vi "Configurations.vi"(8 "Mode":T4) -> (0 "Configuration":T1={"Mode"="", "InstrumentMode"={"MainDAQ_Selector"=enum."None", "LaserCtrlMethod"=enum."SRS_DG535", "InstruMode"=enum."fsLDPI"}, "CommuniationSettings"={"SDG_II"="", "DG535"="", "BNC565"="", "EPM2000"="", "NI-DAQmx"="", "Micos"={"Simulation"=FALSE, "ComPort"="", "Serial Config"={"Baud Rate"=0, "Parity"=0, "Data Bits"=0, "Stop Bits"=0, "Flow Control"=0}, "#Axis"=0}, "ESP300"={"Simulation"=FALSE, "ComPort"="", "Serial Config"={"Baud Rate"=0, "Parity"=0, "Data Bits"=0, "Stop Bits"=0, "Flow Control"=0}, "#Axis"=0}}, "DG535"={"Trigger"={"Trigger Mode"=enum."Internal", "Internal/Burst Rate"=0.0, "External  Level"=0.0, "Impedance"=FALSE, "Slope"=FALSE}, "Delays"=[], "Output"=[]}, "Gage_Config"={"Acquisition"={"Sample Rate"=0.0, "Mode"=0, "Start (0)"=0.0, "Depth"=0.0, "Segment Size"=0.0, "Trigger Delay"=0.0, "Trigger Timeout"=0.0, "Trigger Holdoff"=0.0, "Clock mode"=enum."Internal"}, "Channels"=[], "Trigger"={"Slope"=0, "Level"=0, "Source"=0, "External Range"=0, "External Coupling"=0, "External"=FALSE, "Disable"=FALSE, "External Impedance"=0}, "Mode(Gage)"=enum."Normal"}, "AnalogDisc_Config"={"Acqusition"={"Freq(Hz,SampleRate)"=0.0, "BufferSize"=0, "Mode"=enum."Single", "RecordLength(s)"=0.0}, "Channels"=[], "Trigger"={"TriggerSource"=enum."None", "Timeout(s)"=0.0, "Holdoff(s)"=0.0, "Position/Delay(s)"=0.0}, "AnalogTrigger"={"Channel"=0, "Polarity"=enum."Rising", "Type"=enum."Edge", "Level(V)"=0.0, "Filter"=enum."Decimate", "Hysterisis(V)"=0.0}}, "Micos"={"Velocity"=0.0, "Acceleration"=0.0}, "ESP300"={"Velocity"=[], "Acceleration"=[]}, "EPM2000"={"Factor(A)"=0.0, "Factor(B)"=0.0}, "ProcessMethod"={"TopLine"=0.0, "Threshold"=0.0, "Baseline"=0.0, "ZeroOffset"=0.0, "Processing Mode"=enum."None"}, "Timing(LDPI)"={"Delay(PI)"=0.0, "Delay(Rejection)"=0.0, "NoDelayOffset"=0.0, "RepRate(Hz)"=0.0}, "Cali."=[0.0707, 0.16163, 0.02539], "BNC_Config"={"System"={"Rep.Rate"=1000.0, "Sys Ext Mode"=enum."Triggered", "Mode"=enum."Single Shot"}, "Channels"=[]}} {"Cali." format="%#.6f"; "Timing(LDPI)"."Delay(PI)" format="%#_6p"; "Timing(LDPI)"."Delay(Rejection)" format="%#_6p"; "Timing(LDPI)"."NoDelayOffset" format="%#_6p"; "DG535"."Trigger"."External  Level" min=-2.56 max=2.56 format="%.2f"; "DG535"."Trigger"."Internal/Burst Rate" min=0.001 max=1000000.0 format="%.3f"; "DG535"."Delays"."Delay" format="%#_6p"; "DG535"."Output"."Offset" min=-3.0 max=4.0 format="%.2f"; "DG535"."Output"."Amplitude" min=-3.0 max=4.0 format="%.2f"; "ProcessMethod"."Threshold" format="%#_6p"; "Gage_Config"."Trigger"."External Impedance" items=["50 Ohm", "HiZ"]; "Gage_Config"."Trigger"."External Coupling" items=["DC", "AC"]; "Gage_Config"."Trigger"."External Range" min=2000 max=10000 step=8000; "Gage_Config"."Trigger"."Slope" items=["Rising", "Falling"]; "Gage_Config"."Trigger"."Level" min=-100 max=100; "Gage_Config"."Trigger"."Source" min=0 max=64 step=1; "Gage_Config"."Channels"."Impedance" min=50 max=1000000 step=999950; "Gage_Config"."Channels"."Coupling" items=["DC", "AC"]; "Gage_Config"."Acquisition"."Segment Size" min=256.0 step=128.0; "Gage_Config"."Acquisition"."Trigger Delay" min=0.0 step=128.0; "Gage_Config"."Acquisition"."Trigger Timeout" format="%.0p"; "Gage_Config"."Acquisition"."Trigger Holdoff" min=0.0 step=128.0; "Gage_Config"."Acquisition"."Depth" min=256.0 step=128.0; "Gage_Config"."Acquisition"."Mode" items=["Single", "Dual", "Quad", "Octal"]; "Gage_Config"."Acquisition"."Sample Rate" format="%.0p"; "AnalogDisc_Config"."AnalogTrigger"."Level(V)" format="%#_6p"; "AnalogDisc_Config"."AnalogTrigger"."Hysterisis(V)" format="%#_6p"; "AnalogDisc_Config"."Acqusition"."RecordLength(s)" format="%#_6p"; "AnalogDisc_Config"."Acqusition"."Freq(Hz,SampleRate)" format="%#_6p"; "AnalogDisc_Config"."Trigger"."Position/Delay(s)" format="%#_6p"; "AnalogDisc_Config"."Trigger"."Holdoff(s)" format="%#_6p"; "AnalogDisc_Config"."Trigger"."Timeout(s)" format="%#_6p"})   [LabVIEW 2013]
uses:
  ControlDef/InstrumentConfiguration.ctl
  ControlDef/MainDAQ_Selector.ctl
  ControlDef/LaserCtrl_Method.ctl
  ControlDef/InstruMode_Typedef.ctl
  <instrlib>/DG535/Command/Set Trigger.ctl
  <instrlib>/DG535/Command/DG535_TriggerMode.ctl
  <instrlib>/DG535/Command/Set Delay.ctl
  <instrlib>/DG535/Command/DG535_Channel.ctl
  <instrlib>/DG535/Command/Set Output.ctl
  <instrlib>/DG535/Command/DG535_Output.ctl
  <instrlib>/GageLv_uic/VI/Gage_Configs.ctl
  <instrlib>/AnalogDiscSDKLv/VIs/DWF_AnalogIn_Configurations.ctl
  <instrlib>/AnalogDiscSDKLv/VIs/DWF_AcqMode.ctl
  <instrlib>/AnalogDiscSDKLv/VIs/DWF_Filter.ctl
  <instrlib>/AnalogDiscSDKLv/VIs/DWF_TrigSrc.ctl
  <instrlib>/AnalogDiscSDKLv/VIs/DWF_TrigCond.ctl
  <instrlib>/AnalogDiscSDKLv/VIs/DWF_TrigType.ctl
  ControlDef/ProcessingMode.ctl
  <instrlib>/BNC/Public/BNC_Configs.ctl
  ControlDef/InstrumentSpecificControls/UIC-AToF/InitializationParams_BNC565_2Ch_AToF.ctl
  Hardware/BNC(QuantumComposers)/Command/Set C-Input.ctl
  Hardware/BNC(QuantumComposers)/Command/Set C-Mode.ctl
  Hardware/BNC(QuantumComposers)/Command/Set C-Output.ctl
  Hardware/BNC(QuantumComposers)/Command/Set C-Enable.ctl
  <instrlib>/DG535/SRS_DG535_Lib.lvlib
  <instrlib>/GageLv_uic/Gage.lvlib
  <instrlib>/AnalogDiscSDKLv/AnalogDiscSDKLv.lvlib
panel:
  in  "GetConfigurations":T1[](array[typedef])=[{"Mode"="fsLDPI", "InstrumentMode"={"MainDAQ_Selector"=enum."Gage", "LaserCtrlMethod"=enum."SDG_II", "InstruMode"=enum."fsLDPI"}, "CommuniationSettings"={"SDG_II"="COM6", "DG535"="GPIB0::5::INSTR", "BNC565"="", "EPM2000"="COM5", "NI-DAQmx"="", "Micos"={"Simulation"=FALSE, "ComPort"="COM3", "Serial Config"={"Baud Rate"=115200, "Parity"=0, "Data Bits"=8, "Stop Bits"=10, "Flow Control"=0}, "#Axis"=3}, "ESP300"={"Simulation"=FALSE, "ComPort"="COM7", "Serial Config"={"Baud Rate"=19200, "Parity"=0, "Data Bits"=8, "Stop Bits"=10, "Flow Control"=0}, "#Axis"=3}}, "DG535"={"Trigger"={"Trigger Mode"=enum."External", "Internal/Burst Rate"=10.0, "External  Level"=1.5, "Impedance"=TRUE, "Slope"=FALSE}, "Delays"=[{"Channel"=enum."A Output", "Sync To"=enum."T0 Output", "Delay"=0.0998095}, {"Channel"=enum."B Output", "Sync To"=enum."A Output", "Delay"=2.5e-05}, {"Channel"=enum."C Output", "Sync To"=enum."T0 Output", "Delay"=0.0}, {"Channel"=enum."D Output", "Sync To"=enum."T0 Output", "Delay"=2.3e-05}, {"Channel"=enum."Trigger Input", "Sync To"=enum."T0 Output", "Delay"=0.0}], "Output"=[{"Channel"=enum."A Output", "Level"=enum."TTL", "Load"=TRUE, "Polarity"=TRUE, "Amplitude"=1.0, "Offset"=0.0}, {"Channel"=enum."B Output", "Level"=enum."TTL", "Load"=FALSE, "Polarity"=TRUE, "Amplitude"=1.0, "Offset"=0.0}, {"Channel"=enum."C Output", "Level"=enum."TTL", "Load"=TRUE, "Polarity"=FALSE, "Amplitude"=1.0, "Offset"=0.0}, {"Channel"=enum."D Output", "Level"=enum."TTL", "Load"=TRUE, "Polarity"=FALSE, "Amplitude"=1.0, "Offset"=0.0}, {"Channel"=enum."T0 Output", "Level"=enum."TTL", "Load"=FALSE, "Polarity"=TRUE, "Amplitude"=1.0, "Offset"=0.0}, {"Channel"=enum."AB Output", "Level"=enum."TTL", "Load"=TRUE, "Polarity"=FALSE, "Amplitude"=1.0, "Offset"=0.0}, {"Channel"=enum."CD Output", "Level"=enum."TTL", "Load"=FALSE, "Polarity"=FALSE, "Amplitude"=1.0, "Offset"=0.0}]}, "Gage_Config"={"Acquisition"={"Sample Rate"=500000000.0, "Mode"=0, "Start (0)"=0.0, "Depth"=32768.0, "Segment Size"=32768.0, "Trigger Delay"=0.0, "Trigger Timeout"=-1.0, "Trigger Holdoff"=0.0, "Clock mode"=enum."Internal"}, "Channels"=[{"Coupling"=1, "Differential Input"=FALSE, "Direct-to-ADC"=FALSE, "Range"=2000, "Impedance"=50, "DC Offset"=0, "Filter"=0}], "Trigger"={"Slope"=1, "Level"=25, "Source"=0, "External Range"=10000, "External Coupling"=0, "External"=TRUE, "Disable"=FALSE, "External Impedance"=0}, "Mode(Gage)"=enum."Continuous"}, "AnalogDisc_Config"={"Acqusition"={"Freq(Hz,SampleRate)"=10000000.0, "BufferSize"=8192, "Mode"=enum."Single", "RecordLength(s)"=8192.0}, "Channels"=[], "Trigger"={"TriggerSource"=enum."None", "Timeout(s)"=0.0, "Holdoff(s)"=1e-06, "Position/Delay(s)"=0.0}, "AnalogTrigger"={"Channel"=0, "Polarity"=enum."Rising", "Type"=enum."Pulse", "Level(V)"=0.0, "Filter"=enum."Decimate", "Hysterisis(V)"=0.0}}, "Micos"={"Velocity"=10.0, "Acceleration"=20.0}, "ESP300"={"Velocity"=[0.2, 0.2, 2.0], "Acceleration"=[0.8, 0.8, 0.8]}, "EPM2000"={"Factor(A)"=1.0, "Factor(B)"=1.0}, "ProcessMethod"={"TopLine"=1.0, "Threshold"=0.01, "Baseline"=0.0, "ZeroOffset"=0.0, "Processing Mode"=enum."Drop by Threshold"}, "Timing(LDPI)"={"Delay(PI)"=2.5e-05, "Delay(Rejection)"=-2e-06, "NoDelayOffset"=0.0998095, "RepRate(Hz)"=10.0}, "Cali."=[0.0707, 0.16163, 0.02539], "BNC_Config"={"System"={"Rep.Rate"=1000.0, "Sys Ext Mode"=enum."Triggered", "Mode"=enum."Single Shot"}, "Channels"=[]}}, {"Mode"="nsLDPI", "InstrumentMode"={"MainDAQ_Selector"=enum."Gage", "LaserCtrlMethod"=enum."SDG_II", "InstruMode"=enum."nsLDPI"}, "CommuniationSettings"={"SDG_II"="", "DG535"="GPIB0::5::INSTR", "BNC565"="", "EPM2000"="COM5", "NI-DAQmx"="", "Micos"={"Simulation"=FALSE, "ComPort"="COM3", "Serial Config"={"Baud Rate"=115200, "Parity"=0, "Data Bits"=8, "Stop Bits"=10, "Flow Control"=0}, "#Axis"=3}, "ESP300"={"Simulation"=FALSE, "ComPort"="COM7", "Serial Config"={"Baud Rate"=19200, "Parity"=0, "Data Bits"=8, "Stop Bits"=10, "Flow Control"=0}, "#Axis"=3}}, "DG535"={"Trigger"={"Trigger Mode"=enum."External", "Internal/Burst Rate"=10.0, "External  Level"=1.5, "Impedance"=TRUE, "Slope"=FALSE}, "Delays"=[{"Channel"=enum."A Output", "Sync To"=enum."T0 Output", "Delay"=0.0998095}, {"Channel"=enum."B Output", "Sync To"=enum."A Output", "Delay"=2.5e-05}, {"Channel"=enum."C Output", "Sync To"=enum."T0 Output", "Delay"=0.0}, {"Channel"=enum."D Output", "Sync To"=enum."T0 Output", "Delay"=2.3e-05}, {"Channel"=enum."Trigger Input", "Sync To"=enum."T0 Output", "Delay"=0.0}], "Output"=[{"Channel"=enum."A Output", "Level"=enum."TTL", "Load"=TRUE, "Polarity"=TRUE, "Amplitude"=1.0, "Offset"=0.0}, {"Channel"=enum."B Output", "Level"=enum."TTL", "Load"=FALSE, "Polarity"=TRUE, "Amplitude"=1.0, "Offset"=0.0}, {"Channel"=enum."C Output", "Level"=enum."TTL", "Load"=TRUE, "Polarity"=FALSE, "Amplitude"=1.0, "Offset"=0.0}, {"Channel"=enum."D Output", "Level"=enum."TTL", "Load"=TRUE, "Polarity"=FALSE, "Amplitude"=1.0, "Offset"=0.0}, {"Channel"=enum."T0 Output", "Level"=enum."TTL", "Load"=FALSE, "Polarity"=TRUE, "Amplitude"=1.0, "Offset"=0.0}, {"Channel"=enum."AB Output", "Level"=enum."TTL", "Load"=TRUE, "Polarity"=FALSE, "Amplitude"=1.0, "Offset"=0.0}, {"Channel"=enum."CD Output", "Level"=enum."TTL", "Load"=FALSE, "Polarity"=FALSE, "Amplitude"=1.0, "Offset"=0.0}]}, "Gage_Config"={"Acquisition"={"Sample Rate"=500000000.0, "Mode"=0, "Start (0)"=0.0, "Depth"=32768.0, "Segment Size"=32768.0, "Trigger Delay"=0.0, "Trigger Timeout"=-1.0, "Trigger Holdoff"=0.0, "Clock mode"=enum."Internal"}, "Channels"=[{"Coupling"=1, "Differential Input"=FALSE, "Direct-to-ADC"=FALSE, "Range"=2000, "Impedance"=50, "DC Offset"=0, "Filter"=0}], "Trigger"={"Slope"=1, "Level"=25, "Source"=0, "External Range"=10000, "External Coupling"=0, "External"=TRUE, "Disable"=FALSE, "External Impedance"=0}, "Mode(Gage)"=enum."Continuous"}, "AnalogDisc_Config"={"Acqusition"={"Freq(Hz,SampleRate)"=10000000.0, "BufferSize"=8192, "Mode"=enum."Single", "RecordLength(s)"=8192.0}, "Channels"=[], "Trigger"={"TriggerSource"=enum."None", "Timeout(s)"=0.0, "Holdoff(s)"=1e-06, "Position/Delay(s)"=0.0}, "AnalogTrigger"={"Channel"=0, "Polarity"=enum."Rising", "Type"=enum."Pulse", "Level(V)"=0.0, "Filter"=enum."Decimate", "Hysterisis(V)"=0.0}}, "Micos"={"Velocity"=10.0, "Acceleration"=20.0}, "ESP300"={"Velocity"=[0.2, 0.2, 0.2], "Acceleration"=[0.8, 0.8, 0.8]}, "EPM2000"={"Factor(A)"=1.0, "Factor(B)"=1.0}, "ProcessMethod"={"TopLine"=1.0, "Threshold"=0.01, "Baseline"=0.0, "ZeroOffset"=0.0, "Processing Mode"=enum."Drop by Threshold"}, "Timing(LDPI)"={"Delay(PI)"=2.5e-05, "Delay(Rejection)"=-2e-06, "NoDelayOffset"=0.0001766, "RepRate(Hz)"=10.0}, "Cali."=[0.0707, 0.16163, 0.02539], "BNC_Config"={"System"={"Rep.Rate"=1000.0, "Sys Ext Mode"=enum."Triggered", "Mode"=enum."Single Shot"}, "Channels"=[]}}, {"Mode"="nsLD-fsPI", "InstrumentMode"={"MainDAQ_Selector"=enum."Gage", "LaserCtrlMethod"=enum."SDG_II", "InstruMode"=enum."nsLD-fsPI"}, "CommuniationSettings"={"SDG_II"="COM6", "DG535"="GPIB0::5::INSTR", "BNC565"="", "EPM2000"="COM5", "NI-DAQmx"="", "Micos"={"Simulation"=FALSE, "ComPort"="COM3", "Serial Config"={"Baud Rate"=115200, "Parity"=0, "Data Bits"=8, "Stop Bits"=10, "Flow Control"=0}, "#Axis"=3}, "ESP300"={"Simulation"=FALSE, "ComPort"="COM7", "Serial Config"={"Baud Rate"=19200, "Parity"=0, "Data Bits"=8, "Stop Bits"=10, "Flow Control"=0}, "#Axis"=3}}, "DG535"={"Trigger"={"Trigger Mode"=enum."External", "Internal/Burst Rate"=1000.0, "External  Level"=1.5, "Impedance"=TRUE, "Slope"=FALSE}, "Delays"=[{"Channel"=enum."A Output", "Sync To"=enum."T0 Output", "Delay"=0.0009859}, {"Channel"=enum."B Output", "Sync To"=enum."A Output", "Delay"=-2e-05}, {"Channel"=enum."C Output", "Sync To"=enum."T0 Output", "Delay"=5e-05}, {"Channel"=enum."D Output", "Sync To"=enum."T0 Output", "Delay"=0.000998}, {"Channel"=enum."Trigger Input", "Sync To"=enum."T0 Output", "Delay"=0.0}], "Output"=[{"Channel"=enum."A Output", "Level"=enum."TTL", "Load"=TRUE, "Polarity"=TRUE, "Amplitude"=1.0, "Offset"=0.0}, {"Channel"=enum."B Output", "Level"=enum."TTL", "Load"=TRUE, "Polarity"=TRUE, "Amplitude"=1.0, "Offset"=0.0}, {"Channel"=enum."C Output", "Level"=enum."TTL", "Load"=TRUE, "Polarity"=FALSE, "Amplitude"=1.0, "Offset"=0.0}, {"Channel"=enum."D Output", "Level"=enum."TTL", "Load"=TRUE, "Polarity"=FALSE, "Amplitude"=1.0, "Offset"=0.0}, {"Channel"=enum."T0 Output", "Level"=enum."TTL", "Load"=TRUE, "Polarity"=TRUE, "Amplitude"=1.0, "Offset"=0.0}, {"Channel"=enum."AB Output", "Level"=enum."TTL", "Load"=TRUE, "Polarity"=FALSE, "Amplitude"=1.0, "Offset"=0.0}, {"Channel"=enum."CD Output", "Level"=enum."TTL", "Load"=FALSE, "Polarity"=FALSE, "Amplitude"=1.0, "Offset"=0.0}]}, "Gage_Config"={"Acquisition"={"Sample Rate"=500000000.0, "Mode"=0, "Start (0)"=0.0, "Depth"=32768.0, "Segment Size"=32768.0, "Trigger Delay"=0.0, "Trigger Timeout"=-1.0, "Trigger Holdoff"=0.0, "Clock mode"=enum."Internal"}, "Channels"=[{"Coupling"=1, "Differential Input"=FALSE, "Direct-to-ADC"=FALSE, "Range"=2000, "Impedance"=50, "DC Offset"=0, "Filter"=0}], "Trigger"={"Slope"=1, "Level"=25, "Source"=0, "External Range"=10000, "External Coupling"=0, "External"=TRUE, "Disable"=FALSE, "External Impedance"=0}, "Mode(Gage)"=enum."Continuous"}, "AnalogDisc_Config"={"Acqusition"={"Freq(Hz,SampleRate)"=10000000.0, "BufferSize"=8192, "Mode"=enum."Single", "RecordLength(s)"=8192.0}, "Channels"=[], "Trigger"={"TriggerSource"=enum."None", "Timeout(s)"=0.0, "Holdoff(s)"=1e-06, "Position/Delay(s)"=0.0}, "AnalogTrigger"={"Channel"=0, "Polarity"=enum."Rising", "Type"=enum."Edge", "Level(V)"=0.0, "Filter"=enum."Decimate", "Hysterisis(V)"=0.0}}, "Micos"={"Velocity"=10.0, "Acceleration"=20.0}, "ESP300"={"Velocity"=[0.2, 0.2, 2.0], "Acceleration"=[0.8, 0.8, 0.8]}, "EPM2000"={"Factor(A)"=1.0, "Factor(B)"=1.0}, "ProcessMethod"={"TopLine"=1.0, "Threshold"=0.01, "Baseline"=0.0, "ZeroOffset"=0.0, "Processing Mode"=enum."Drop by Threshold"}, "Timing(LDPI)"={"Delay(PI)"=2.5e-05, "Delay(Rejection)"=-2e-06, "NoDelayOffset"=0.0009859, "RepRate(Hz)"=1000.0}, "Cali."=[0.0707, 0.16163, 0.02539], "BNC_Config"={"System"={"Rep.Rate"=1000.0, "Sys Ext Mode"=enum."Triggered", "Mode"=enum."Single Shot"}, "Channels"=[]}}, {"Mode"="GenericTOF", "InstrumentMode"={"MainDAQ_Selector"=enum."Gage", "LaserCtrlMethod"=enum."BNC", "InstruMode"=enum."GenericTOF"}, "CommuniationSettings"={"SDG_II"="", "DG535"="", "BNC565"="COM4", "EPM2000"="", "NI-DAQmx"="", "Micos"={"Simulation"=FALSE, "ComPort"="COM3", "Serial Config"={"Baud Rate"=57600, "Parity"=0, "Data Bits"=8, "Stop Bits"=10, "Flow Control"=0}, "#Axis"=3}, "ESP300"={"Simulation"=TRUE, "ComPort"="", "Serial Config"={"Baud Rate"=19200, "Parity"=0, "Data Bits"=8, "Stop Bits"=10, "Flow Control"=0}, "#Axis"=3}}, "DG535"={"Trigger"={"Trigger Mode"=enum."Internal", "Internal/Burst Rate"=200.0, "External  Level"=1.5, "Impedance"=TRUE, "Slope"=FALSE}, "Delays"=[], "Output"=[]}, "Gage_Config"={"Acquisition"={"Sample Rate"=200000000.0, "Mode"=0, "Start (0)"=0.0, "Depth"=16384.0, "Segment Size"=16384.0, "Trigger Delay"=0.0, "Trigger Timeout"=-1.0, "Trigger Holdoff"=0.0, "Clock mode"=enum."Internal"}, "Channels"=[{"Coupling"=0, "Differential Input"=FALSE, "Direct-to-ADC"=FALSE, "Range"=2000, "Impedance"=50, "DC Offset"=0, "Filter"=0}], "Trigger"={"Slope"=1, "Level"=25, "Source"=0, "External Range"=10000, "External Coupling"=0, "External"=TRUE, "Disable"=FALSE, "External Impedance"=0}, "Mode(Gage)"=enum."Continuous"}, "AnalogDisc_Config"={"Acqusition"={"Freq(Hz,SampleRate)"=10000000.0, "BufferSize"=8192, "Mode"=enum."Single", "RecordLength(s)"=8192.0}, "Channels"=[], "Trigger"={"TriggerSource"=enum."None", "Timeout(s)"=0.0, "Holdoff(s)"=1e-06, "Position/Delay(s)"=0.0}, "AnalogTrigger"={"Channel"=0, "Polarity"=enum."Rising", "Type"=enum."Pulse", "Level(V)"=0.0, "Filter"=enum."Decimate", "Hysterisis(V)"=0.0}}, "Micos"={"Velocity"=10.0, "Acceleration"=20.0}, "ESP300"={"Velocity"=[], "Acceleration"=[]}, "EPM2000"={"Factor(A)"=1.0, "Factor(B)"=1.0}, "ProcessMethod"={"TopLine"=1.0, "Threshold"=0.01, "Baseline"=0.0, "ZeroOffset"=0.0, "Processing Mode"=enum."Drop by Threshold"}, "Timing(LDPI)"={"Delay(PI)"=0.0, "Delay(Rejection)"=0.0, "NoDelayOffset"=0.0, "RepRate(Hz)"=50.0}, "Cali."=[0.0, 1.0, 0.0], "BNC_Config"={"System"={"Rep.Rate"=1000.0, "Sys Ext Mode"=enum."Triggered", "Mode"=enum."Single Shot"}, "Channels"=[]}}, {"Mode"="BeamProfiling", "InstrumentMode"={"MainDAQ_Selector"=enum."AnalogDisc", "LaserCtrlMethod"=enum."SRS_DG535", "InstruMode"=enum."GenericTOF"}, "CommuniationSettings"={"SDG_II"="", "DG535"="GPIB0::5::INSTR", "BNC565"="", "EPM2000"="", "NI-DAQmx"="", "Micos"={"Simulation"=TRUE, "ComPort"="", "Serial Config"={"Baud Rate"=57600, "Parity"=0, "Data Bits"=8, "Stop Bits"=10, "Flow Control"=0}, "#Axis"=3}, "ESP300"={"Simulation"=FALSE, "ComPort"="COM1", "Serial Config"={"Baud Rate"=19200, "Parity"=0, "Data Bits"=8, "Stop Bits"=10, "Flow Control"=0}, "#Axis"=3}}, "DG535"={"Trigger"={"Trigger Mode"=enum."External", "Internal/Burst Rate"=50.0, "External  Level"=1.5, "Impedance"=TRUE, "Slope"=FALSE}, "Delays"=[], "Output"=[]}, "Gage_Config"={"Acquisition"={"Sample Rate"=125000000.0, "Mode"=0, "Start (0)"=0.0, "Depth"=16384.0, "Segment Size"=16384.0, "Trigger Delay"=0.0, "Trigger Timeout"=-1.0, "Trigger Holdoff"=0.0, "Clock mode"=enum."Internal"}, "Channels"=[{"Coupling"=1, "Differential Input"=FALSE, "Direct-to-ADC"=FALSE, "Range"=2000, "Impedance"=50, "DC Offset"=0, "Filter"=0}], "Trigger"={"Slope"=1, "Level"=25, "Source"=0, "External Range"=10000, "External Coupling"=0, "External"=TRUE, "Disable"=FALSE, "External Impedance"=0}, "Mode(Gage)"=enum."Continuous"}, "AnalogDisc_Config"={"Acqusition"={"Freq(Hz,SampleRate)"=10000000.0, "BufferSize"=8192, "Mode"=enum."Single", "RecordLength(s)"=8192.0}, "Channels"=[{"Range(V)"=5.0, "Offset(V)"=0.0, "Filter"=enum."Average", "Enable"=TRUE}], "Trigger"={"TriggerSource"=enum."DetectorAnalogIn", "Timeout(s)"=0.0, "Holdoff(s)"=1e-06, "Position/Delay(s)"=0.0}, "AnalogTrigger"={"Channel"=0, "Polarity"=enum."Rising", "Type"=enum."Edge", "Level(V)"=0.0, "Filter"=enum."Average", "Hysterisis(V)"=0.0}}, "Micos"={"Velocity"=10.0, "Acceleration"=20.0}, "ESP300"={"Velocity"=[0.2, 0.2, 0.2], "Acceleration"=[0.8, 0.8, 0.8]}, "EPM2000"={"Factor(A)"=1.0, "Factor(B)"=1.0}, "ProcessMethod"={"TopLine"=1.0, "Threshold"=0.01, "Baseline"=0.0, "ZeroOffset"=0.0, "Processing Mode"=enum."None"}, "Timing(LDPI)"={"Delay(PI)"=0.0, "Delay(Rejection)"=0.0, "NoDelayOffset"=0.0, "RepRate(Hz)"=50.0}, "Cali."=[0.0, 1.0, 0.0], "BNC_Config"={"System"={"Rep.Rate"=1000.0, "Sys Ext Mode"=enum."Triggered", "Mode"=enum."Single Shot"}, "Channels"=[]}}] {"Cali." format="%#.6f"; "Timing(LDPI)"."Delay(PI)" format="%#_6p"; "Timing(LDPI)"."Delay(Rejection)" format="%#_6p"; "Timing(LDPI)"."NoDelayOffset" format="%#_6p"; "DG535"."Trigger"."External  Level" min=-2.56 max=2.56 format="%.2f"; "DG535"."Trigger"."Internal/Burst Rate" min=0.001 max=1000000.0 format="%.3f"; "DG535"."Delays"."Delay" format="%#_6p"; "DG535"."Output"."Offset" min=-3.0 max=4.0 format="%.2f"; "DG535"."Output"."Amplitude" min=-3.0 max=4.0 format="%.2f"; "ProcessMethod"."Threshold" format="%#_6p"; "Gage_Config"."Trigger"."External Impedance" items=["50 Ohm", "HiZ"]; "Gage_Config"."Trigger"."External Coupling" items=["DC", "AC"]; "Gage_Config"."Trigger"."External Range" min=2000 max=10000 step=8000; "Gage_Config"."Trigger"."Slope" items=["Rising", "Falling"]; "Gage_Config"."Trigger"."Level" min=-100 max=100; "Gage_Config"."Trigger"."Source" min=0 max=64 step=1; "Gage_Config"."Channels"."Impedance" min=50 max=1000000 step=999950; "Gage_Config"."Channels"."Coupling" items=["DC", "AC"]; "Gage_Config"."Acquisition"."Segment Size" min=256.0 step=128.0; "Gage_Config"."Acquisition"."Trigger Delay" min=0.0 step=128.0; "Gage_Config"."Acquisition"."Trigger Timeout" format="%.0p"; "Gage_Config"."Acquisition"."Trigger Holdoff" min=0.0 step=128.0; "Gage_Config"."Acquisition"."Depth" min=256.0 step=128.0; "Gage_Config"."Acquisition"."Mode" items=["Single", "Dual", "Quad", "Octal"]; "Gage_Config"."Acquisition"."Sample Rate" format="%.0p"; "AnalogDisc_Config"."AnalogTrigger"."Level(V)" format="%#_6p"; "AnalogDisc_Config"."AnalogTrigger"."Hysterisis(V)" format="%#_6p"; "AnalogDisc_Config"."Acqusition"."RecordLength(s)" format="%#_6p"; "AnalogDisc_Config"."Acqusition"."Freq(Hz,SampleRate)" format="%#_6p"; "AnalogDisc_Config"."Trigger"."Position/Delay(s)" format="%#_6p"; "AnalogDisc_Config"."Trigger"."Holdoff(s)" format="%#_6p"; "AnalogDisc_Config"."Trigger"."Timeout(s)" format="%#_6p"}
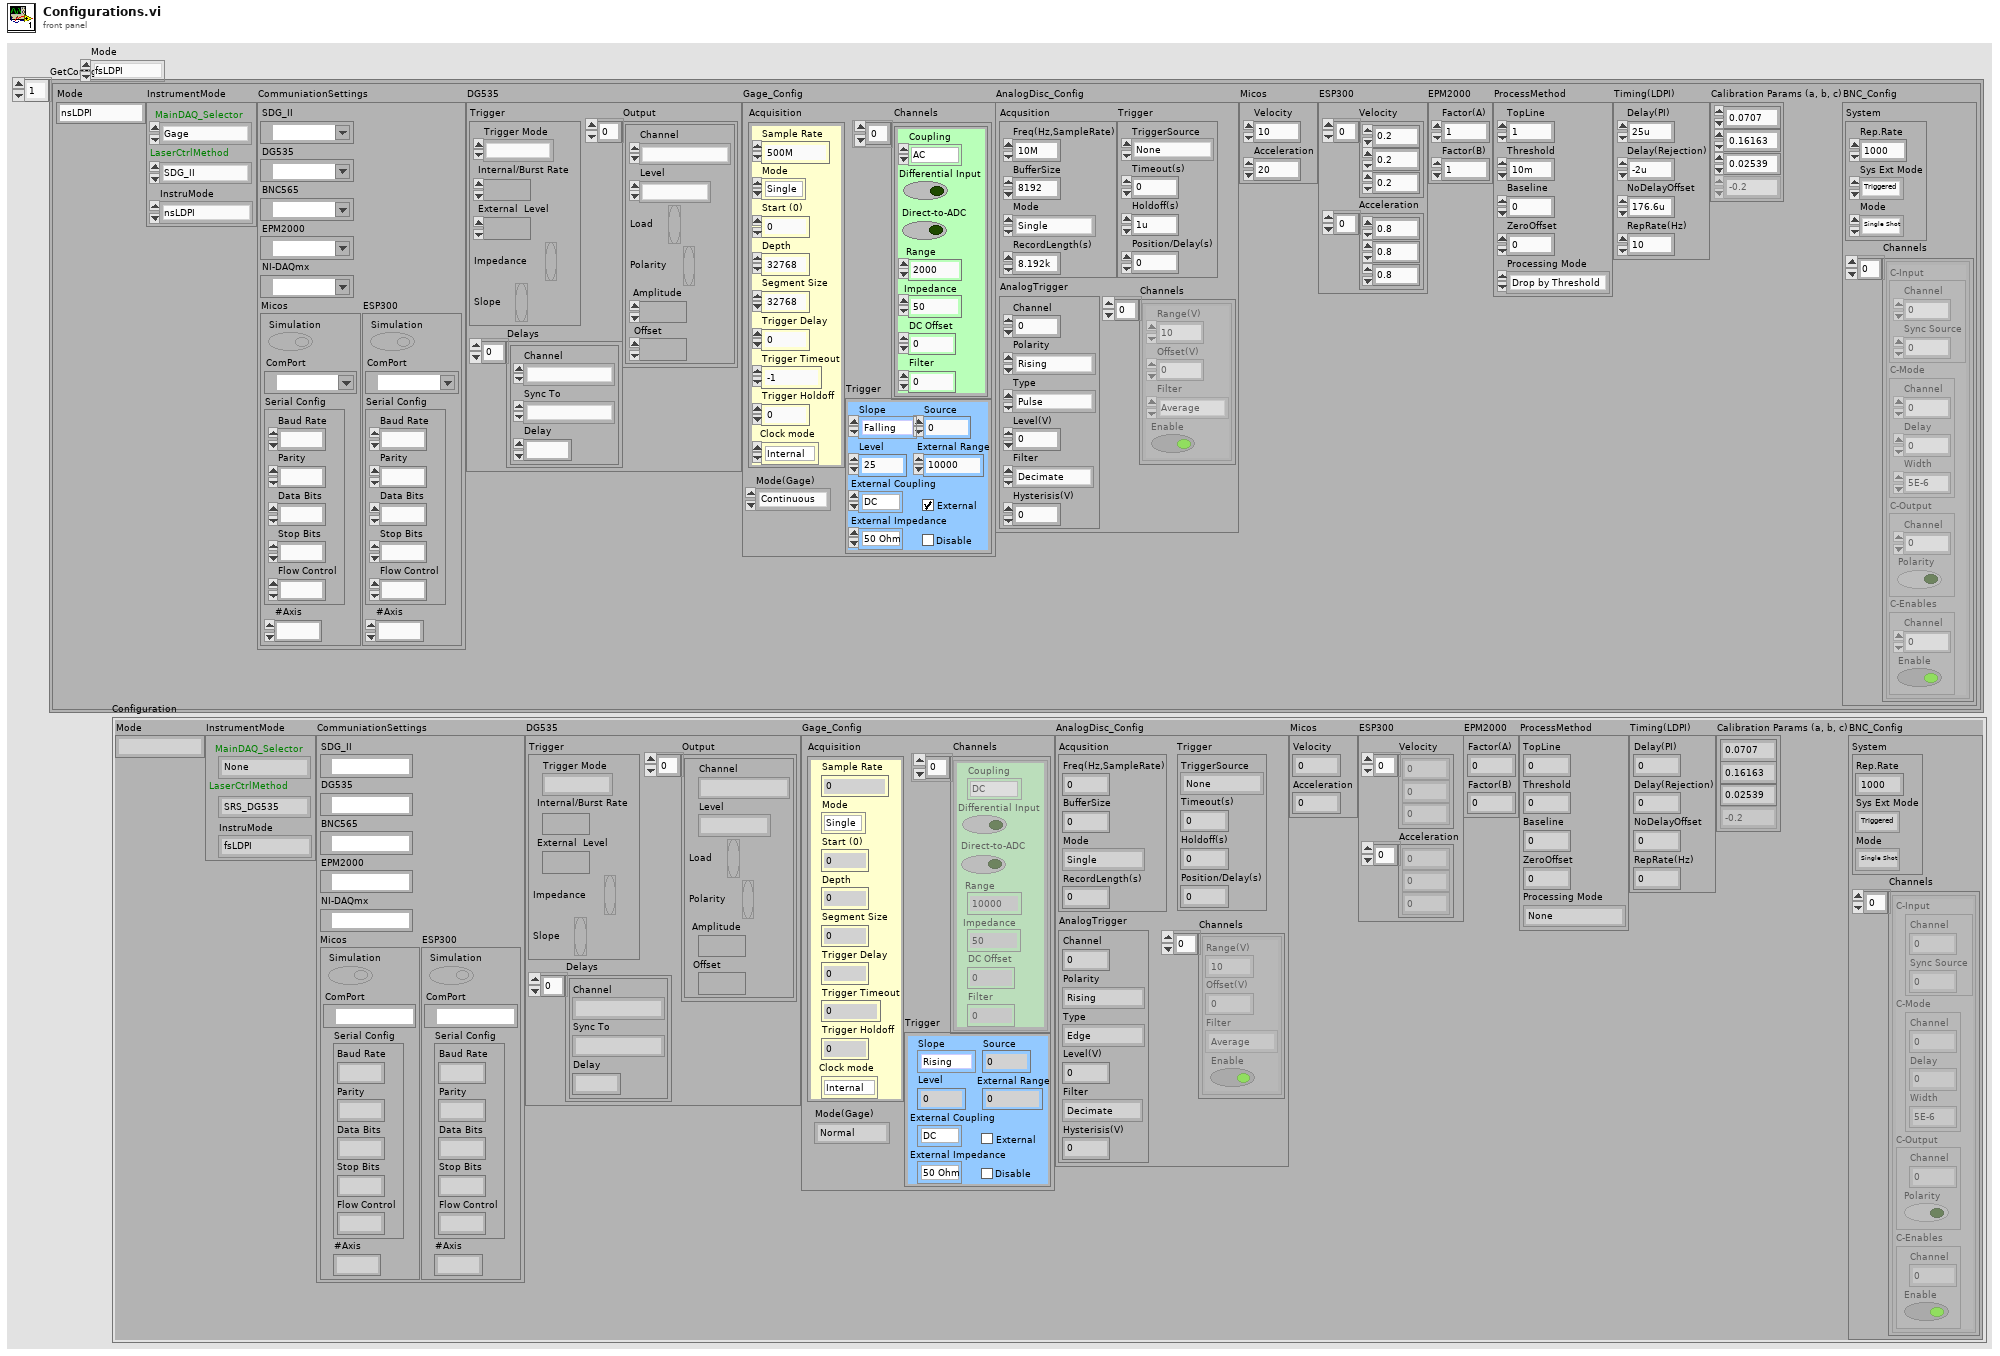
[diagram p1: front panel]
types:
  T1 = typedef "InstrumentConfiguration.ctl" = cluster{"Mode":string, "InstrumentMode":cluster{"MainDAQ_Selector":T2, "LaserCtrlMethod":T3, "InstruMode":T4}, "CommuniationSettings":cluster{"SDG_II":refnum<visa-resource-name>, "DG535":refnum<visa-resource-name>, "BNC565":refnum<visa-resource-name>, "EPM2000":refnum<visa-resource-name>, "NI-DAQmx":refnum<visa-resource-name>, "Micos":cluster{"Simulation":bool, "ComPort":refnum<visa-resource-name>, "Serial Config":cluster{"Baud Rate":u32, "Parity":u16, "Data Bits":u16, "Stop Bits":u16, "Flow Control":u16}, "#Axis":i32}, "ESP300":cluster{"Simulation":bool, "ComPort":refnum<visa-resource-name>, "Serial Config":cluster{"Baud Rate":u32, "Parity":u16, "Data Bits":u16, "Stop Bits":u16, "Flow Control":u16}, "#Axis":i32}}, "DG535":cluster{"Trigger":T5, "Delays":T7[], "Output":T9[]}, "Gage_Config":T11, "AnalogDisc_Config":T12, "Micos":cluster{"Velocity":dbl, "Acceleration":dbl}, "ESP300":cluster{"Velocity":dbl[], "Acceleration":dbl[]}, "EPM2000":cluster{"Factor(A)":dbl, "Factor(B)":dbl}, "ProcessMethod":cluster{"TopLine":dbl, "Threshold":dbl, "Baseline":dbl, "ZeroOffset":dbl, "Processing Mode":T18}, "Timing(LDPI)":cluster{"Delay(PI)":dbl, "Delay(Rejection)":dbl, "NoDelayOffset":dbl, "RepRate(Hz)":dbl}, "Cali.":dbl[], "BNC_Config":T19}
  T2 = typedef "MainDAQ_Selector.ctl" = enum16{"None", "Gage", "Gage_Double", "IonWerks_TDCx4", "Tektronics", "KnifeEdge_Emu", "AnalogDisc"}
  T3 = typedef "LaserCtrl_Method.ctl" = enum16{"SRS_DG535", "BNC", "SDG_II"}
  T4 = typedef "InstruMode_Typedef.ctl" = enum16{"fsLDPI", "nsLDPI", "nsLD-fsPI", "GenericTOF", "BeamProfiling"}
  T5 = typedef "SRS_DG535_Lib.lvlib/Set Trigger.ctl" = cluster{"Trigger Mode":T6, "Internal/Burst Rate":dbl, "External  Level":sgl, "Impedance":bool, "Slope":bool}
  T6 = typedef "SRS_DG535_Lib.lvlib/DG535_TriggerMode.ctl" = enum16{"Internal", "External", "SingleShot", "Burst", "Line"}
  T7 = typedef "SRS_DG535_Lib.lvlib/Set Delay.ctl" = cluster{"Channel":T8, "Sync To":T8, "Delay":dbl}
  T8 = typedef "SRS_DG535_Lib.lvlib/DG535_Channel.ctl" = enum16{"Trigger Input", "T0 Output", "A Output", "B Output", "AB Output", "C Output", "D Output", "CD Output", "NULL"}
  T9 = typedef "SRS_DG535_Lib.lvlib/Set Output.ctl" = cluster{"Channel":T8, "Level":T10, "Load":bool, "Polarity":bool, "Amplitude":dbl, "Offset":dbl}
  T10 = typedef "SRS_DG535_Lib.lvlib/DG535_Output.ctl" = enum16{"TTL", "NIM", "ECL", "Variable"}
  T11 = typedef "Gage.lvlib/Gage_Configs.ctl" = cluster{"Acquisition":cluster{"Sample Rate":dbl, "Mode":u16, "Start (0)":dbl, "Depth":dbl, "Segment Size":dbl, "Trigger Delay":dbl, "Trigger Timeout":dbl, "Trigger Holdoff":dbl, "Clock mode":enum16{"Internal", "External", "Reference"}}, "Channels":cluster{"Coupling":u16, "Differential Input":bool, "Direct-to-ADC":bool, "Range":u32, "Impedance":u32, "DC Offset":i32, "Filter":i32}[], "Trigger":cluster{"Slope":u16, "Level":i32, "Source":i32, "External Range":u32, "External Coupling":u16, "External":bool, "Disable":bool, "External Impedance":u16}, "Mode(Gage)":enum16{"Normal", "Continuous", "MultiRecord", "HwAverage"}}
  T12 = typedef "AnalogDiscSDKLv.lvlib/DWF_AnalogIn_Configurations.ctl" = cluster{"Acqusition":cluster{"Freq(Hz,SampleRate)":dbl, "BufferSize":i32, "Mode":T13, "RecordLength(s)":dbl}, "Channels":cluster{"Range(V)":dbl, "Offset(V)":dbl, "Filter":T14, "Enable":bool}[], "Trigger":cluster{"TriggerSource":T15, "Timeout(s)":dbl, "Holdoff(s)":dbl, "Position/Delay(s)":dbl}, "AnalogTrigger":cluster{"Channel":i32, "Polarity":T16, "Type":T17, "Level(V)":dbl, "Filter":T14, "Hysterisis(V)":dbl}}
  T13 = typedef "AnalogDiscSDKLv.lvlib/DWF_AcqMode.ctl" = enum16{"Single", "ScanShift", "ScanScreen", "Record"}
  T14 = typedef "AnalogDiscSDKLv.lvlib/DWF_Filter.ctl" = enum16{"Decimate", "Average", "MinMax"}
  T15 = typedef "AnalogDiscSDKLv.lvlib/DWF_TrigSrc.ctl" = enum16{"None", "PC", "DetectorAnalogIn", "DetectorDigitalIn", "AnalogIn", "DigitalIn", "DigitalOut", "AnalogOut1", "AnalogOut2", "AnalogOut3", "AnalogOut4", "External1", "External2", "External3", "External4"}
  T16 = typedef "AnalogDiscSDKLv.lvlib/DWF_TrigCond.ctl" = enum16{"Rising", "Falling"}
  T17 = typedef "AnalogDiscSDKLv.lvlib/DWF_TrigType.ctl" = enum16{"Edge", "Pulse", "Transition"}
  T18 = typedef "ProcessingMode.ctl" = enum16{"None", "Drop by Threshold", "TDC Simulate", "SetFilter"}
  T19 = typedef "BNC_Configs.ctl" = cluster{"System":cluster{"Rep.Rate":dbl, "Sys Ext Mode":enum16{"Disabled", "Triggered", "Gated", "Triggered & Gated"}, "Mode":enum16{"Normal", "Single Shot", "Duty Cycle", "Burst"}}, "Channels":T20[]}
  T20 = typedef "InitializationParams_BNC565_2Ch_AToF.ctl" = cluster{"C-Input":T21, "C-Mode":T22, "C-Output":T23, "C-Enables":T24}
  T21 = typedef "Set C-Input.ctl" = cluster{"Channel":i32, "Sync Source":i32}
  T22 = typedef "Set C-Mode.ctl" = cluster{"Channel":i32, "Delay":dbl, "Width":dbl}
  T23 = typedef "Set C-Output.ctl" = cluster{"Channel":i32, "Polarity":bool}
  T24 = typedef "Set C-Enable.ctl" = cluster{"Channel":i32, "Enable":bool}
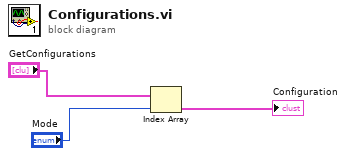
[diagram p0: block diagram]
diagram:
  n1 = Index Array(array="GetConfigurations", index="Mode") -> (element=→"Configuration":T1)
